vi "SQL Time to Timestamp.vi"(1 "Get:Get String":string) -> (0 "Time Stamp":timestamp)   [LabVIEW 2013, in "Data.PGSQL.lvclass"]
uses:
  Data.PGSQL.lvclass
panel:
  out "error out":errorcluster
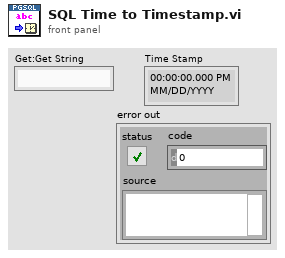
[diagram p1: front panel]
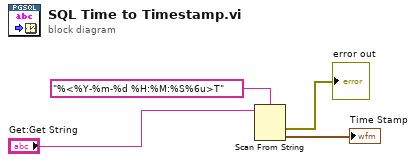
[diagram p0: block diagram]
diagram:
  n1 = Scan From String(format string="%<%Y-%m-%d %H:%M:%S%6u>T", input string="Get:Get String") -> (error out=→"error out":errorcluster, output 1=→"Time Stamp":timestamp)  [unwired: 3 in, 2 out]
